vi "WPI_RobotDriveDelayAndUpdateSafety.vi"(6 "Feed time (s)":dbl=0.05, 8 "error in (no error)":errorcluster, 10 "Delay (s)":dbl, 11 "RobotDriveDevRef":T1={"DevStatus"={"status"=FALSE, "code"=0, "source"=""}, "Motors[]"=[], "Square Inputs"=FALSE, "Max Output"=1.0}) -> (0 "error out":errorcluster, 3 "RobotDriveDevRef 2":T1={"DevStatus"={"status"=FALSE, "code"=0, "source"=""}, "Motors[]"=[], "Square Inputs"=FALSE, "Max Output"=1.0})   [LabVIEW 2025]
doc: "During autonomous, it is often useful to update motor speed, then delay before updating them again. This delay uses the refnum to easily sequence the operations, and it updates the safety mechanism so that the drive motors are not disabled.\n\nThis software is licensed. Open the labview\\readme\\WPI Robotics Library Open Source License.txt file for more information."
uses:
  <vilib>/Rock Robotics/WPI/RobotDrive/WPI_RobotDriveDevRef.ctl
  <vilib>/Rock Robotics/WPI/MotorControl/WPI_MotorControlDeviceRef.ctl
  <vilib>/Rock Robotics/WPI/MotorControl/WPI_MotorControlType.ctl
  <vilib>/Rock Robotics/SystemInterfaces/DIO/FPGA_DIOPWMChannel.ctl
  <vilib>/Rock Robotics/WPI/PWM/WPI_PWMDeadband.ctl
  <vilib>/Rock Robotics/SystemInterfaces/DIO/FPGA_DIOChannel.ctl
  <vilib>/Rock Robotics/WPI/RobotDrive/WPI_RobotDriveSafetyCheck.vi
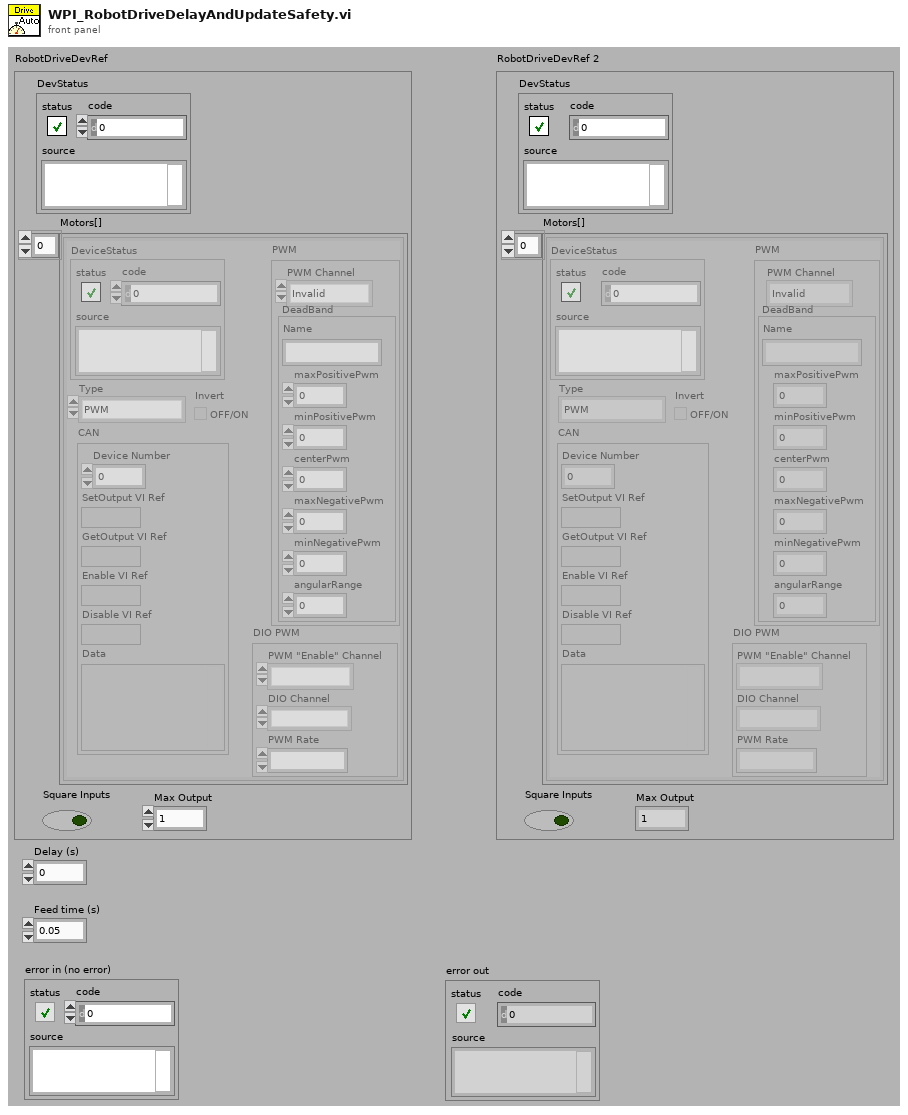
[diagram p1: front panel]
types:
  T1 = typedef "WPI_RobotDriveDevRef.ctl" = cluster{"DevStatus":errorcluster, "Motors[]":T2[], "Square Inputs":bool, "Max Output":dbl}
  T2 = typedef "WPI_MotorControlDeviceRef.ctl" = cluster{"DeviceStatus":errorcluster, "Type":T3, "PWM":cluster{"PWM Channel":T4, "DeadBand":T5}, "CAN":cluster{"Device Number":u8, "SetOutput VI Ref":variant, "GetOutput VI Ref":variant, "Enable VI Ref":variant, "Disable VI Ref":variant, "Data":variant}, "Invert":bool, "DIO PWM":cluster{"PWM \"Enable\" Channel":T4, "DIOChannel":T6, "PWM Rate":dbl}}
  T3 = typedef "WPI_MotorControlType.ctl" = enum16{"PWM", "CAN", "DIO PWM"}
  T4 = typedef "FPGA_DIOPWMChannel.ctl" = enum8{"PWM 0", "PWM 1", "PWM 2", "PWM 3", "PWM 4", "PWM 5", "PWM 6", "PWM 7", "PWM 8", "PWM 9", "PWM MXP 0", "PWM MXP 1", "PWM MXP 2", "PWM MXP 3", "PWM MXP 4", "PWM MXP 5", "PWM MXP 6", "PWM MXP 7", "PWM MXP 8", "PWM MXP 9", "Invalid"}
  T5 = typedef "WPI_PWMDeadband.ctl" = cluster{"Name":string, "maxPositivePwm":i32, "minPositivePwm":i32, "centerPwm":i32, "maxNegativePwm":i32, "minNegativePwm":i32, "angularRange":u16}
  T6 = typedef "FPGA_DIOChannel.ctl" = enum8{"DIO 0", "DIO 1", "DIO 2", "DIO 3", "DIO 4", "DIO 5", "DIO 6", "DIO 7", "DIO 8", "DIO 9", "DIO MXP 0", "DIO MXP 1", "DIO MXP 2", "DIO MXP 3", "DIO MXP 4", "DIO MXP 5", "DIO MXP 6", "DIO MXP 7", "DIO MXP 8", "DIO MXP 9", "DIO MXP 10", "DIO MXP 11", "DIO MXP 12", "DIO MXP 13", "DIO MXP 14", "DIO MXP 15", "SPI Port CS1", "SPI Port CS2", "SPI Port CS3", "SPI Port MISO", "SPI Port MOSI", "Invalid"}
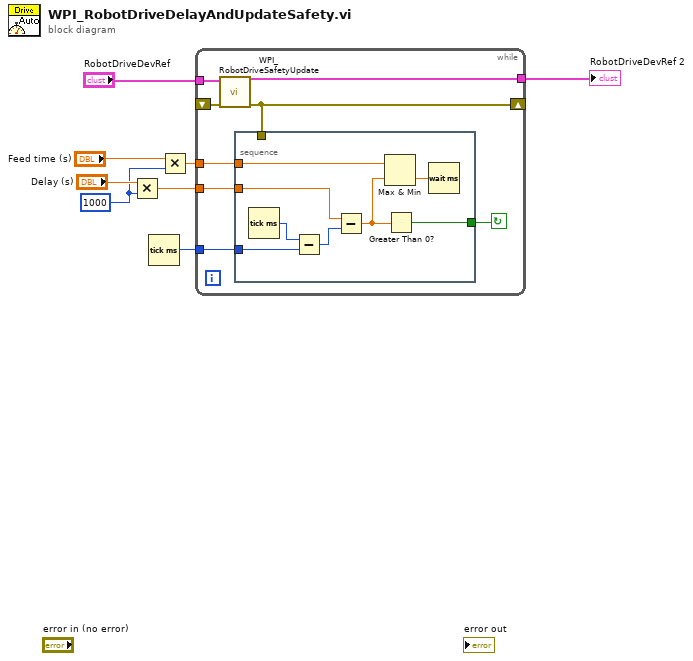
[diagram p0: block diagram]
diagram:
  w1 = 1000
  n1 = Multiply(x="Delay (s)", y=w1) -> (x*y=w4:dbl)
  n2 = Tick Count (ms)() -> (millisecond timer value=w6:u32)
  n3 = Multiply(x="Feed time (s)", y=w1) -> (x*y=w5:dbl)
  n4 = while {
    tunnel: w4 -> [w14]
    tunnel: [w12] -> w7
    shift-right: [w9] -> _
    shift-left: _ -> [w10]
    tunnel: w5 -> [w15]
    tunnel: w6 -> [w16]
    tunnel: "RobotDriveDevRef" -> [w11]
    stop <- w13 continue-if-true
    n5 = call <vilib>:"WPI_RobotDriveSafetyUpdate.vi"("error in (no error)"=w10, "RobotDriveDevRef"=w11) -> ("error out"=w9:errorcluster, "RobotDriveDevRef"=w12:T1)  [unwired: 8 out]
    n6 = stacked-sequence {
      tunnel: w16 -> [w24]
      tunnel: w15 -> [w23]
      tunnel: w14 -> [w21]
      tunnel: w9 -> [_]
      tunnel: [w17] -> w13
      frame #0 {
        n7 = Tick Count (ms)() -> (millisecond timer value=w19:u32)
        n8 = Subtract(x=w19, y=w24) -> (x-y=w20:u32)
        n9 = Subtract(x=w21, y=w20) -> (x-y=w18:dbl)
        n10 = Max & Min(x=w23, y=w18) -> (min(x,y)=w22:dbl)  [unwired: 1 out]
        n11 = Greater Than 0?(x=w18) -> (x > 0?=w17:bool)
        n12 = Wait (ms)(milliseconds to wait=w22) -> ()  [unwired: 1 out]
      }
    }
  }
  "RobotDriveDevRef 2" <- w7
